vi "Pigeon2_open.vi"(10 "CANbus Name":string="rio", 11 "Device ID":u8) -> (3 "DeviceReference 2":T1)   [LabVIEW 2023]
uses:
  Users/Cory/Documents/PhoenixPro-LabVIEW-Generation/controls/DeviceReference.ctl
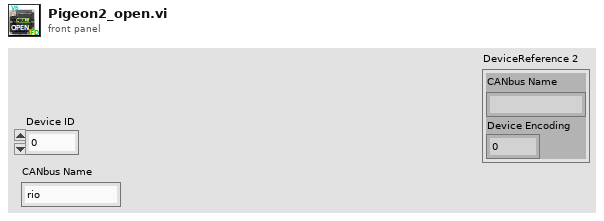
[diagram p1: front panel]
types:
  T1 = typedef "DeviceReference.ctl" = cluster{"CANbus Name":string, "Device Encoding":u32}
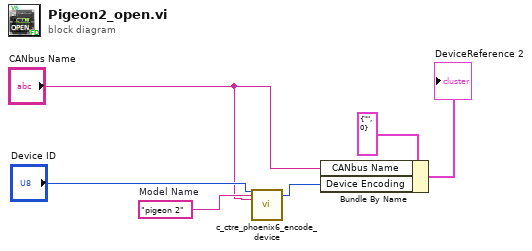
[diagram p0: block diagram]
diagram:
  w2 = "pigeon 2"  # Model Name
  n1 = call <vilib>:"c_ctre_phoenix6_encode_device.vi"("Numeric 2"="Device ID", "String"=w2, "String 2"="CANbus Name") -> ("Numeric 3"=w3:u32)  [unwired: 23 in, 1 out]
  n2 = Bundle By Name(cluster=T1 {"CANbus Name"="", "Device Encoding"=0} ("DeviceReference"), "CANbus Name"="CANbus Name", "Device Encoding"=w3) -> (→"DeviceReference 2":T1)
